vi "Write Data2D.lvclass.vi"(8 "error in (no error)":errorcluster, 10 "Data2D.lvclass":refnum<class "Data2D.lvclass">, 11 "Experiment2D in":refnum<class "Experiment2D.lvclass">) -> (0 "error out":errorcluster, 3 "Experiment2D out":refnum<class "Experiment2D.lvclass">)   [LabVIEW 2018, in "Experiment2D.lvclass"]
uses:
  Experiment2D.lvclass
  Data/Data2D/Data2D.lvclass
  Experiment2D.lvclass/Experiment2D.ctl
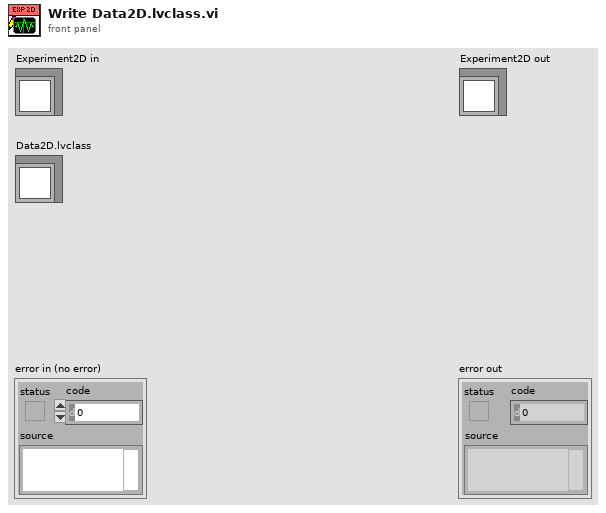
[diagram p1: front panel]
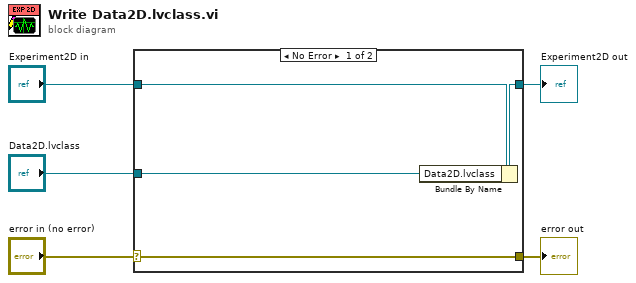
[diagram p0: block diagram]
diagram:
  n1 = case shown="No Error" "error in (no error)" {
    selector: "error in (no error)" -> [w9 w10]
    tunnel: [w9 w10] -> w4
    tunnel: [w7 w11] -> w2
    tunnel: "Experiment2D in" -> [w8 w11]
    tunnel: "Data2D.lvclass" -> [w6 _]
    frame No Error {
      n2 = Bundle By Name(cluster=w8, "Data2D.lvclass"=w6) -> (w7:refnum<class "Experiment2D.lvclass">)
    }
    frame Error {
    }
  }
  "error out" <- w4
  "Experiment2D out" <- w2
